vi "CreateFileIVPath.vi"(8 "error in":errorcluster, 11 "File Name":string) -> (0 "error out":errorcluster, 3 "appended path":path)   [LabVIEW 2020, in "SMU.lvclass"]
uses:
  SMU/SMU.lvclass
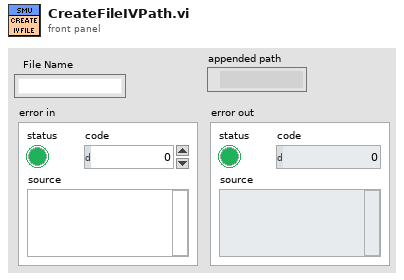
[diagram p1: front panel]
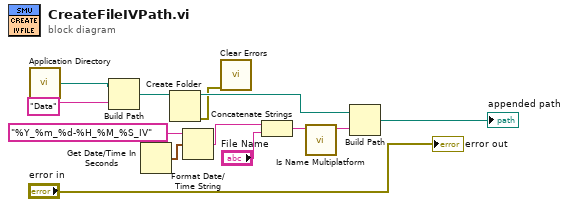
[diagram p0: block diagram]
diagram:
  n1 = call <vilib>:"Application Directory.vi"() -> ("Application Directory"=w10:path)
  n2 = Build Path(base path=w10, name or relative path="Data") -> (appended path=w3:path)
  n3 = Get Date/Time In Seconds() -> (seconds since 1Jan1904=w6:timestamp)
  n4 = Create Folder(path (use dialog)=w3) -> (created path=w2:path, error out=w1:errorcluster)  [unwired: 2 in, 1 out]
  n5 = Format Date/Time String(time format string (%c)="%Y_%m_%d-%H_%M_%S_IV", seconds (now)=w6) -> (date/time string=w12:string)  [unwired: 1 in]
  n6 = call <vilib>:"Clear Errors.vi"("error in (no error)"=w1) -> ()  [unwired: 5 in, 2 out]
  n7 = Concatenate Strings(w12, "File Name") -> (w8:string)
  n8 = call <vilib>:"Is Name Multiplatform.vi"("filename"=w8) -> ("suggested filename"=w7:string)  [unwired: 6 in, 4 out]
  n9 = Build Path(base path=w2, name or relative path=w7) -> (appended path=→"appended path":path)
  "error out" <- "error in"
